vi "SQLite DB Path.vi"(9 "Password":string, 10 "ping":bool, 11 "database":string="database1.db") -> (3 "Path out":string)   [LabVIEW 2016, in "SQLite Lib.lvlib"]
uses:
  SQLite Lib.lvlib
  <vilib>/Utility/sysdir.llb/System Directory Type.ctl
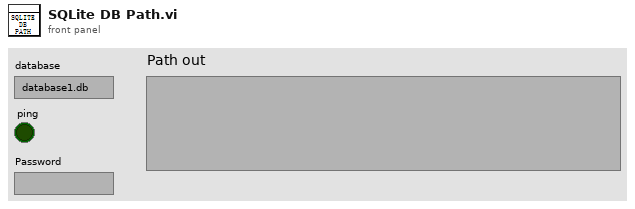
[diagram p1: front panel]
types:
  T1 = typedef "System Directory Type.ctl" = i32
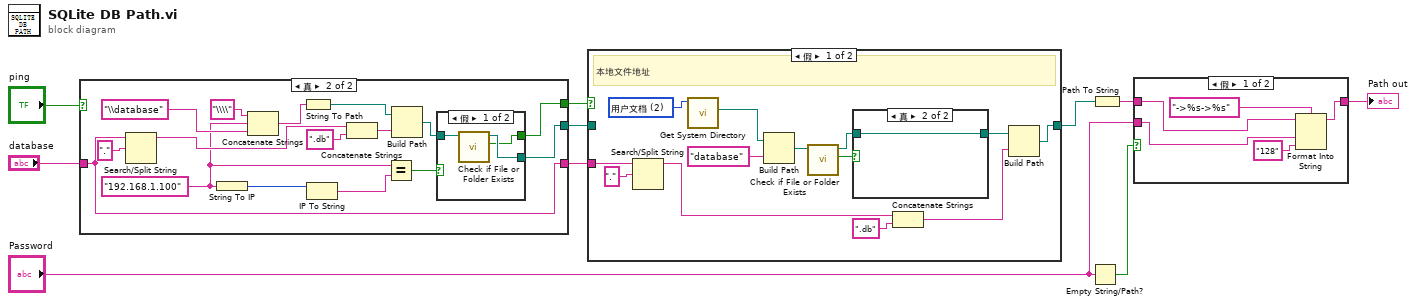
[diagram p0: block diagram]
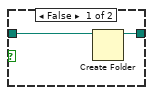
[diagram p3: hidden frame]
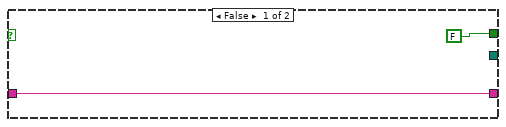
[diagram p5: hidden frame]
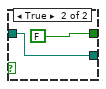
[diagram p6: hidden frame]
diagram:
  n1 = case shown="真" "ping" {
    tunnel: [_ w22] -> w6
    tunnel: [FALSE ("file or folder exists?") w21] -> w8
    tunnel: [w11 w16] -> w7
    tunnel: "database" -> [w11 w16]
    frame False {
    }
    frame True {
      w13 = "192.168.1.100" ("名称")
      n2 = Search/Split String(string=w16, search string/char (-)="." ("搜索字符串/字符(-)")) -> (substring before match=w20:string)  [unwired: 1 in, 2 out]
      n3 = String To IP(1:w13) -> (0:w28:u32)
      n4 = Concatenate Strings("\\\\" ("字符串"), w13, "\\database" ("名称或相对路径")) -> (w26:string)
      n5 = String To Path(string=w26) -> (path=w14:path)
      n6 = IP To String(2:w28) -> (0:w25:string)  [unwired: 1 in]
      n7 = Concatenate Strings(w20, ".db" ("字符串")) -> (w17:string)
      n8 = Equal?(x=w13, y=w25) -> (x = y?=w24:bool)
      n9 = Build Path(base path=w14, name or relative path=w17) -> (appended path=w23:path)
      n10 = case shown="假" w24 {
        tunnel: w23 -> [w31 w32]
        tunnel: [w30 w32] -> w22
        tunnel: [w29 FALSE] -> w21
        frame False {
          n11 = call <vilib>:"Check if File or Folder Exists.vi"("path"=w31) -> ("file or folder exists?"=w29:bool, "dup path"=w30:path)  [unwired: 8 in, 1 out]
        }
        frame True {
        }
      }
    }
  }
  n12 = case shown="假" w8 {
    tunnel: [w46 w50] -> w4
    tunnel: w7 -> [w34 _]
    tunnel: w6 -> [_ w50]
    frame False {
      w38 = T1 2 items=["用户目录"=0, "用户桌面"=1, "用户文档"=2, "用户应用程序数据"=3, "用户设置"=4, "用户临时目录"=5, "公共文档"=6, "公共应用程序数据"=7, "公共设置"=8, "公共缓存"=13, "系统核心库"=9, "系统安装库"=10, "应用程序文件"=11, "启动盘根目录"=12] ("system directory type")
      # "本地文件地址"
      n13 = Search/Split String(string=w34, search string/char (-)="." ("搜索字符串/字符(-)")) -> (substring before match=w42:string)  [unwired: 1 in, 2 out]
      n14 = call <vilib>:"Get System Directory.vi"("system directory type"=w38) -> ("system directory"=w37:path)  [unwired: 10 in]
      n15 = Build Path(base path=w37, name or relative path="database" ("名称或相对路径")) -> (appended path=w35:path)
      n16 = call <vilib>:"Check if File or Folder Exists.vi"("path"=w35) -> ("file or folder exists?"=w45:bool, "dup path"=w44:path)  [unwired: 8 in, 1 out]
      n17 = case shown="真" w45 {
        tunnel: w44 -> [w48 w49]
        tunnel: [w47 w49] -> w43
        frame False {
          n18 = Create Folder(path (use dialog)=w48) -> (created path=w47:path)  [unwired: 2 in, 2 out]
        }
        frame True {
        }
      }
      n19 = Concatenate Strings(w42, ".db" ("字符串")) -> (w41:string)
      n20 = Build Path(base path=w43, name or relative path=w41) -> (appended path=w46:path)
    }
    frame True {
    }
  }
  n21 = Empty String/Path?(string/path="Password") -> (empty?=w1:bool)
  n22 = Path To String(path=w4) -> (string=w5:string)
  n23 = case shown="假" w1 {
    tunnel: w5 -> [w54 w56]
    tunnel: [w53 w56] -> w3
    tunnel: "Password" -> [w51 _]
    frame False {
      n24 = Format Into String(format string="->%s->%s", initial string=w54, w51, "128" ("Enter Password")) -> (resulting string=w53:string)  [unwired: 1 in, 1 out]
    }
    frame True {
    }
  }
  "Path out" <- w3
